vi "Test_StructureSubdiagramsAndDeleteObject.vi"() -> ()   [LabVIEW 2025]
uses:
  8cebb4ce-4f0f-4319-9f7e-82e401bee674.vi
  ff6ee880-e87d-4ac2-b0b9-a7c0f406254d.vi
  57ba1f44-eecb-4af5-975d-0cda700306c1.vi
  Scripting Server.lvlib
panel:
  out "result":string
  out "error out":errorcluster
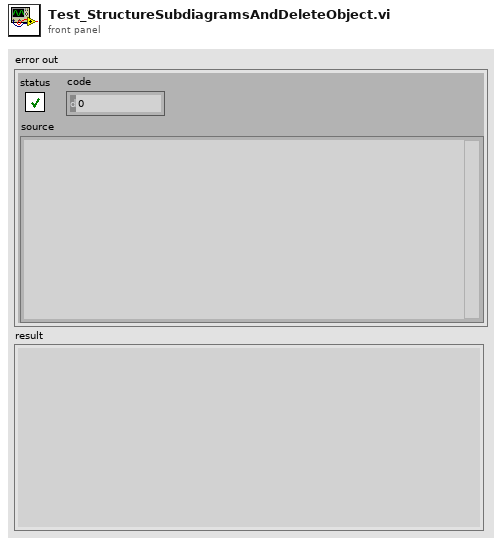
[diagram p1: front panel]
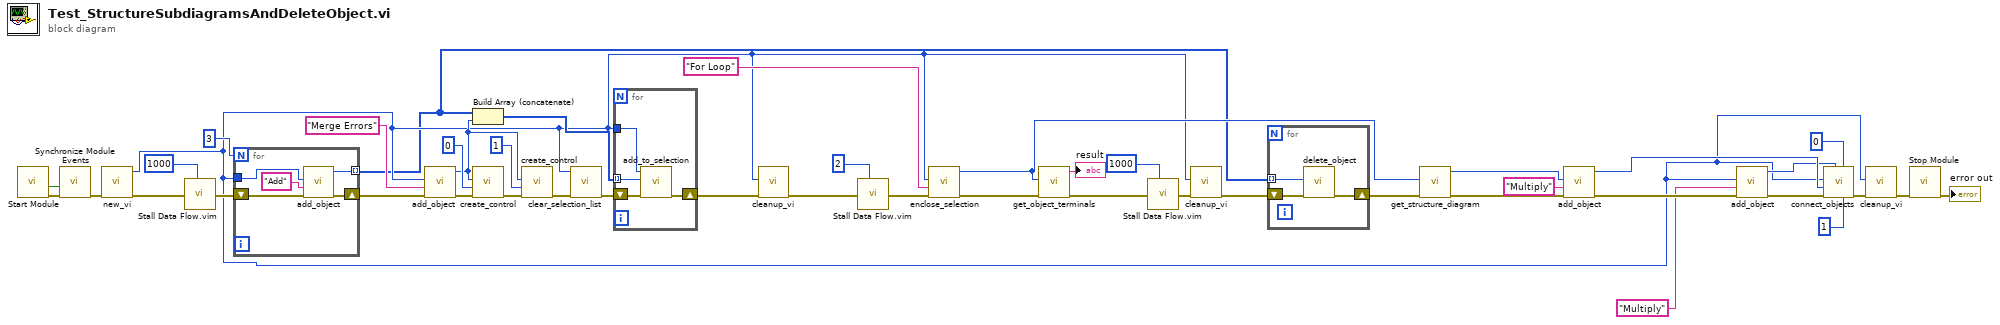
[diagram p0: block diagram]
diagram:
  n1 = call "Start Module.vi"() -> ("error out"=w44:errorcluster, "Wait for Event Sync?"=w45:bool)  [unwired: 7 in, 3 out]
  n2 = call "Synchronize Module Events.vi"("error in"=w44, "Wait for Event Sync?"=w45) -> ("error out"=w43:errorcluster)  [unwired: 9 in]
  n3 = call "new_vi.vi"("error in"=w43) -> ("error out"=w42:errorcluster, "vi_id"=w2:i32)  [unwired: 7 in, 2 out]
  n4 = call "Stall Data Flow.vim"("value in"=w42, "milliseconds to wait"=u32 1000) -> ("value out"=w41:errorcluster)  [unwired: 1 out]
  n5 = for {
    N: 3 -> [_]
    shift-right: [w49] -> w39
    shift-left: w41 -> [w50]
    tunnel: w2 -> [w46]
    tunnel: [w48] -> w1 mode=indexing
    n6 = call "add_object.vi"("error in"=w50, "object_name"="Add", "diagram_id"=w46) -> ("error out"=w49:errorcluster, "object_id"=w48:i32)  [unwired: 5 in, 2 out]
  }
  n7 = call "add_object.vi"("error in"=w39, "object_name"="Merge Errors", "diagram_id"=w2) -> ("error out"=w34:errorcluster, "object_id"=w26:i32)  [unwired: 5 in, 2 out]
  n8 = Build Array (concatenate)(w1, w26) -> (w16:i32[])
  n9 = call "create_control.vi"("error in"=w34, "terminal_index"=0, "object_id"=w26) -> ("error out"=w32:errorcluster)  [unwired: 6 in, 2 out]
  n10 = call "create_control.vi"("error in"=w32, "terminal_index"=1, "object_id"=w26) -> ("error out"=w30:errorcluster)  [unwired: 6 in, 2 out]
  n11 = call "clear_selection_list.vi"("error in"=w30, "vi_id"=w2) -> ("error out"=w28:errorcluster)  [unwired: 8 in, 1 out]
  n12 = for {
    tunnel: w2 -> [w52]
    tunnel: w16 -> [w51] mode=indexing
    shift-right: [w53] -> w27
    shift-left: w28 -> [w54]
    n13 = call "add_to_selection.vi"("error in"=w54, "object_id"=w51, "vi_id"=w52) -> ("error out"=w53:errorcluster)  [unwired: 7 in, 1 out]
  }
  n14 = call "cleanup_vi.vi"("error in"=w27, "vi_reference"=w2) -> ("error out"=w20:errorcluster)  [unwired: 7 in, 2 out]
  n15 = call "Stall Data Flow.vim"("value in"=w20, "milliseconds to wait"=u32 2) -> ("value out"=w23:errorcluster)  [unwired: 1 out]
  n16 = call "enclose_selection.vi"("error in"=w23, "structure_type"="For Loop", "vi_id"=w2) -> ("error out"=w25:errorcluster, "object_id"=w14:i32)  [unwired: 6 in, 1 out]
  n17 = call "get_object_terminals.vi"("error in"=w25, "object_id"=w14) -> ("error out"=w19:errorcluster, "result"=→"result":string)  [unwired: 7 in, 1 out]
  n18 = call "Stall Data Flow.vim"("value in"=w19, "milliseconds to wait"=u32 1000) -> ("value out"=w38:errorcluster)  [unwired: 1 out]
  n19 = call "cleanup_vi.vi"("error in"=w38, "vi_reference"=w2) -> ("error out"=w36:errorcluster)  [unwired: 7 in, 2 out]
  n20 = for {
    tunnel: w1 -> [w55] mode=indexing
    shift-right: [w56] -> w17
    shift-left: w36 -> [w57]
    n21 = call "delete_object.vi"("error in"=w57, "object_id"=w55) -> ("error out"=w56:errorcluster)  [unwired: 8 in, 1 out]
  }
  n22 = call "get_structure_diagram.vi"("error in"=w17, "structure_id"=w14) -> ("error out"=w15:errorcluster, "diagram_id"=w12:i32)  [unwired: 7 in, 1 out]
  n23 = call "add_object.vi"("error in"=w15, "object_name"="Multiply", "diagram_id"=w12) -> ("error out"=w13:errorcluster, "object_id"=w7:i32)  [unwired: 5 in, 2 out]
  n24 = call "add_object.vi"("error in"=w13, "object_name"="Multiply", "diagram_id"=w2) -> ("error out"=w10:errorcluster, "object_id"=w6:i32)  [unwired: 5 in, 2 out]
  n25 = call "connect_objects.vi"("to_object_terminal_index"=1 ("from_object_terminal_index"), "from_object_terminal_index"=0, "to_object_reference"=w6, "error in"=w10, "from_object_reference"=w7, "vi_reference"=w2) -> ("error out"=w8:errorcluster)  [unwired: 3 in, 2 out]
  n26 = call "cleanup_vi.vi"("error in"=w8, "vi_reference"=w2) -> ("error out"=w3:errorcluster)  [unwired: 7 in, 2 out]
  n27 = call "Stop Module.vi"("error in"=w3) -> ("error out"=→"error out":errorcluster)  [unwired: 10 in]
